vi "feed_forward.vi"(4 "Weights Cluster":cluster{"Array":dbl[][]}[](array[cluster]), 7 "Input Data":dbl[][](array[numeric]), 10 "act":bool, 11 "# hidden layers":i32) -> (6 "Neurons":cluster{"Array":cluster{"Array 2":dbl[]}[]}[](array[cluster]))   [LabVIEW 2016]
uses:
  <vilib>/Analysis/baseanly.llb/Vector x A.vi
  <vilib>/Analysis/NI_AALBase.lvlib
panel:
  # "Feed Forward unit"
  # "Author: Adam Cavatassi, McGill University, 2018"
  # "Inputs"
  # "Outputs"
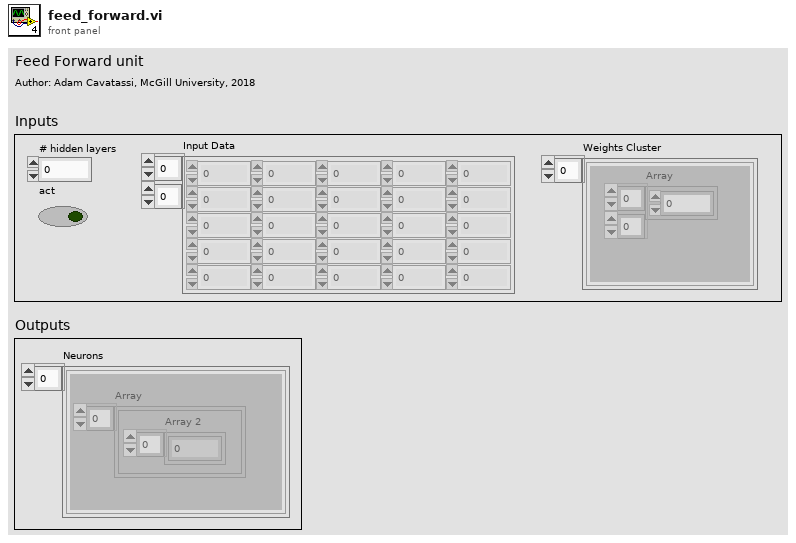
[diagram p1: front panel]
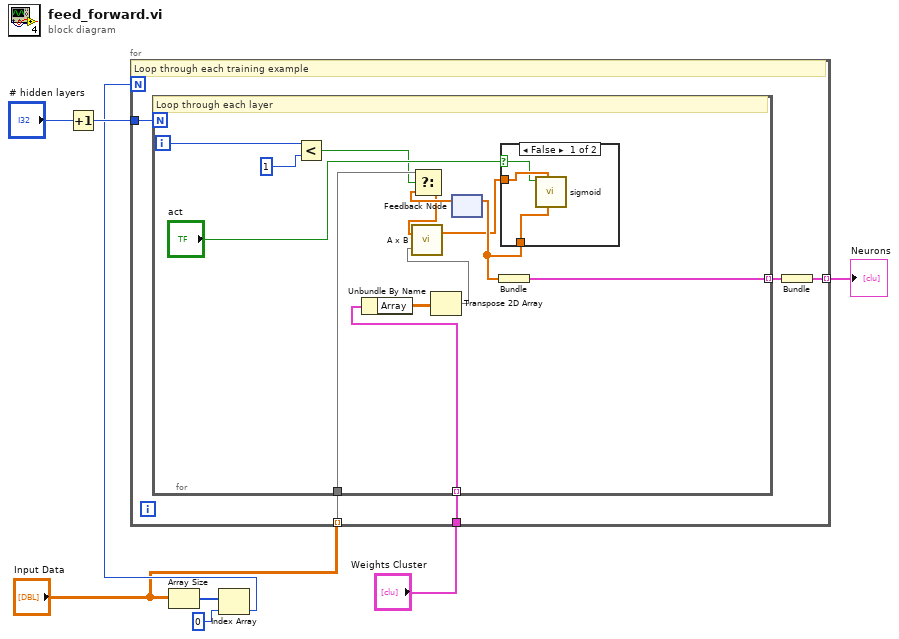
[diagram p0: block diagram]
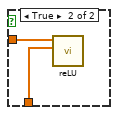
[diagram p2: hidden frame]
diagram:
  n1 = Increment(x="# hidden layers") -> (x+1=w8:i32)
  n2 = Array Size(array="Input Data") -> (size(s)=w7:i32[])
  n3 = Index Array(array=w7, index=0) -> (element=w5:i32)
  n4 = for {
    N: w5 -> [_]
    tunnel: w8 -> [w11]
    tunnel: "Weights Cluster" -> [w12]
    tunnel: "Input Data" -> [w13] mode=indexing
    tunnel: [w9] -> w1 mode=indexing
    # "Loop through each training example"
    n5 = for {
      N: w11 -> [_]
      tunnel: w12 -> [w24] mode=indexing
      tunnel: w13 -> [w25]
      tunnel: [w23] -> w10 mode=indexing
      i -> [w26]
      # "Loop through each layer"
      n6 = Less?(x=w26, y=1) -> (x < y?=w19:bool)
      n7 = Unbundle By Name(w24) -> ("Array"=w16:dbl[][])
      n8 = Transpose 2D Array(2D array=w16) -> (transposed array=w20:dbl[][])
      n9 = feedback #1() -> (w18:dbl[])  [unwired: 1 in]
      n10 = Select(t=w25, s=w19, f=w18) -> (s? t:f=w17:dbl[])
      n11 = call-poly <vilib>:"A x B.vi"("Matrix A"=w20, "Vector V'"=w17) -> ("V' x A"=w14:dbl[])  [unwired: 1 out]
      n12 = case shown="False" "act" {
        selector: "act" -> [w27 _]
        tunnel: [w28 w31] -> w15
        tunnel: w14 -> [w29 w30]
        frame False {
          n13 = call "sigmoid.vi"("Input"=w29, "Derivative?"=w27) -> ("Output"=w28:dbl[])  [unwired: 9 in]
        }
        frame True {
          n14 = call "reLU.vi"("Input"=w30) -> ("Output"=w31:dbl[])  [unwired: 10 in]
        }
      }
      n15 = feedback-in #1(w15) -> ()
      n16 = Bundle("Output"=w15) -> (w23:cluster{"Output":dbl[]})  [unwired: 1 in]
    }
    n17 = Bundle(w10) -> (w9:cluster{cluster{"Output":dbl[]}[]})  [unwired: 1 in]
  }
  "Neurons" <- w1
